vi "Tab Render.vi"(6 "Offset X (1)":i16=1, 7 "Mouse Coords":T2, 8 "error in (no error)":errorcluster, 9 "Active Idx (-1)":i32=-1, 10 "Tab Symbols":i32[](array[numeric]), 11 "Tab Names":string[](array[string])) -> (0 "error out":errorcluster, 1 "Tab X Rects":T1(array[cluster]), 2 "Tab Rects":T1(array[cluster]), 3 "Picture":picture)   [LabVIEW 2018, in "Tab.lvlib"]
uses:
  Tab.lvlib
  Theme/Theme Colors.vi
  Theme/Theme.lvlib
  <vilib>/Utility/miscctls.llb/LVPoint32TypeDef.ctl
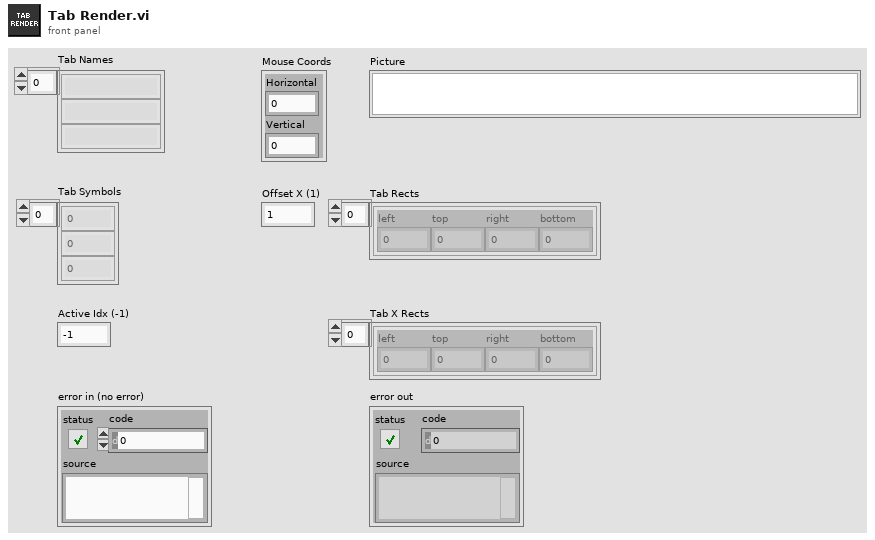
[diagram p1: front panel]
types:
  T1 = cluster{"left":i16, "top":i16, "right":i16, "bottom":i16}[]
  T2 = typedef "LVPoint32TypeDef.ctl" = cluster{"Horizontal":i32, "Vertical":i32}
  T3 = cluster{"Font Name:":string, "Size":i16, "Strikeout?":bool, "Italic?":bool, "Underline?":bool, "Outline?":bool, "Shadow?":bool, "Bold?":bool}
  T4 = enum16{"User-specified Font", "Application Font", "System Font", "Dialog Font"}
  T5 = cluster{"left":i16, "top":i16, "right":i16, "bottom":i16}
  T6 = typedef "imagedata.ctl" = cluster{"image type":i32, "image depth":i32, "image":u8[], "mask":u8[], "colors":u32[], "Rectangle":cluster{"left":i16, "top":i16, "right":i16, "bottom":i16}}
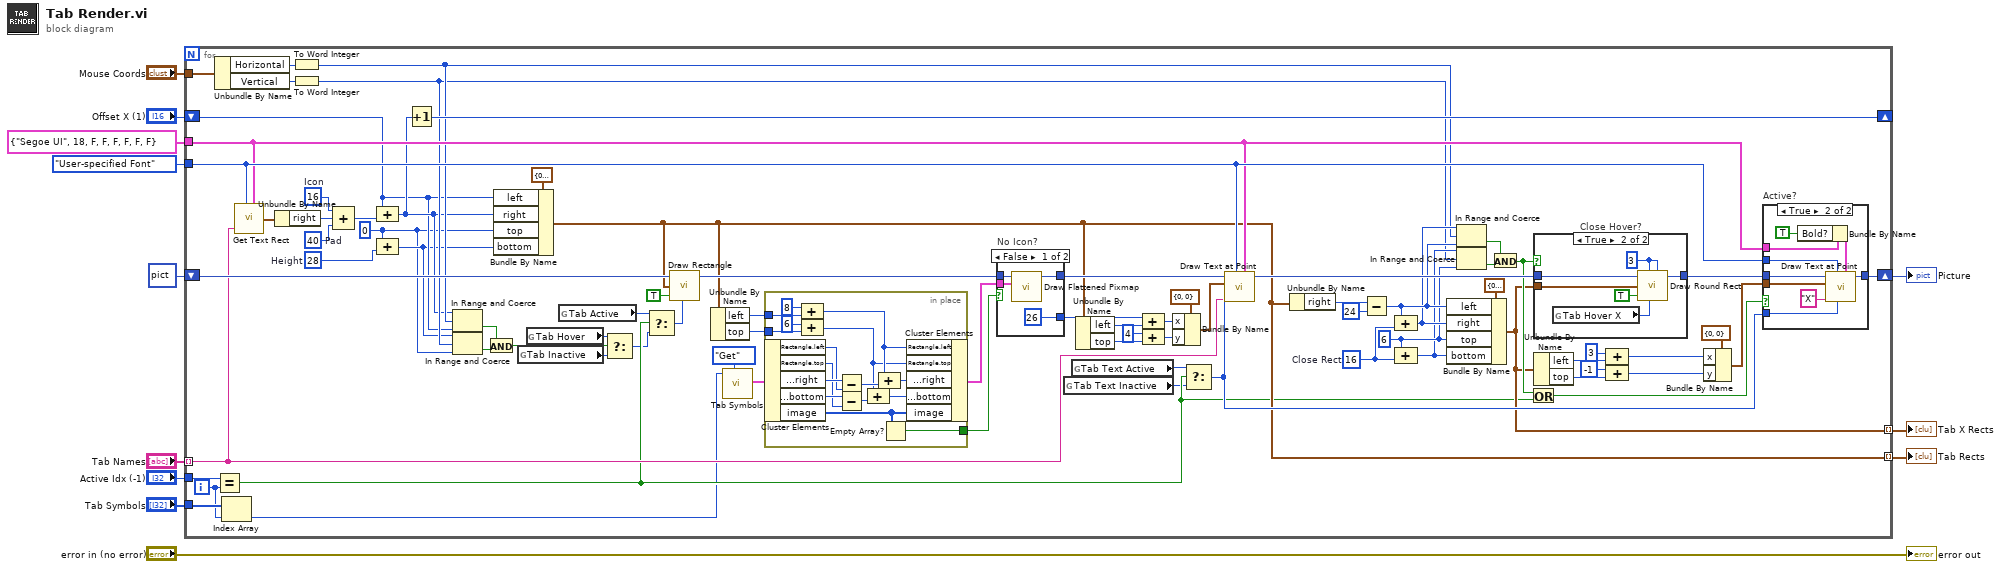
[diagram p0: block diagram]
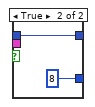
[diagram p2: hidden frame]
diagram:
  n1 = for {
    tunnel: "Tab Names" -> [w38] mode=indexing
    tunnel: T4."User-specified Font" ("desired font(Application)") -> [w50]
    tunnel: T3 {"Font Name:"="Segoe UI", "Size"=18, "Strikeout?"=FALSE, "Italic?"=FALSE, "Underline?"=FALSE, "Outline?"=FALSE, "Shadow?"=FALSE, "Bold?"=FALSE} ("[user-specified font]") -> [w49]
    shift-right: [w88] -> w2
    shift-left: picture data[5B] ("new picture") -> [w74]
    shift-right: [w82] -> _
    shift-left: "Offset X (1)" -> [w20]
    tunnel: "Mouse Coords" -> [w40]
    tunnel: [w36] -> w7 mode=indexing
    tunnel: [w35] -> w6 mode=indexing
    tunnel: "Active Idx (-1)" -> [w34]
    tunnel: "Tab Symbols" -> [w32]
    i -> [w31]
    w58 = i16 16  # Close Rect
    w42 = i16 6 ("top")
    w75 = i16 28  # Height
    w18 = i16 0 ("top")
    w78 = i16 40  # Pad
    w79 = i16 16  # Icon
    n2 = Unbundle By Name(w40) -> ("Horizontal"=w48:i32, "Vertical"=w47:i32)
    n3 = Equal?(x=w34, y=w31) -> (x = y?=w33:bool)
    n4 = Index Array(array=w32, index=w31) -> (element=w30:i32)
    n5 = call <vilib>:"Get Text Rect.vi"("desired font(Application)"=w50, "text"=w38, "[user-specified font]"=w49) -> ("rect"=w81:T5)  [unwired: 6 in]
    n6 = Unbundle By Name(w81) -> ("right"=w80:i16)
    n7 = To Word Integer(number=w48) -> (16bit integer=w23:i16)
    n8 = To Word Integer(number=w47) -> (16bit integer=w22:i16)
    n9 = Compound Arithmetic op=ADD(w79, w80, w78) -> (w76:i16)
    n10 = Compound Arithmetic op=ADD(w20, w76) -> (w21:i16)
    n11 = Compound Arithmetic op=unknown(w18, w75) -> (w19:i16)
    n12 = Increment(x=w21) -> (x+1=w82:i16)
    n13 = In Range and Coerce(upper limit=w21, x=w23, lower limit=w20) -> (In Range?=w26:bool)  [unwired: 1 out]
    n14 = In Range and Coerce(upper limit=w19, x=w22, lower limit=w18) -> (In Range?=w24:bool)  [unwired: 1 out]
    n15 = And(x=w26, y=w24) -> (x .and. y?=w25:bool)
    n16 = Bundle By Name(cluster=T5 {"left"=0, "top"=0, "right"=0, "bottom"=0} ("y"), "left"=w20, "right"=w21, "top"=w18, "bottom"=w19) -> (w36:T5)
    n17 = global read "Theme Colors.vi" "Tab Inactive"() -> (w16:u32)
    n18 = global read "Theme Colors.vi" "Tab Hover"() -> (w17:u32)
    n19 = global read "Theme Colors.vi" "Tab Active"() -> (w15:u32)
    n20 = Select(t=w17, s=w25, f=w16) -> (s? t:f=w27:u32)
    n21 = Select(t=w15, s=w33, f=w27) -> (s? t:f=w87:u32)
    n22 = call <vilib>:"Draw Rectangle.vi"("picture"=w74, "rect"=w36, "fill?(F)"=TRUE, "color(black)"=w87) -> ("new picture"=w73:picture)  [unwired: 5 in]
    n23 = Unbundle By Name(w36) -> ("left"=w70:i16, "top"=w71:i16)
    n24 = call "Tab Symbols.vi"("Action (Get)"=enum8{"Get", "Set"}."Get", "Symbol Idx"=w30) -> ("Symbol Image out"=w29:T6)  [unwired: 7 in, 2 out]
    n25 = in-place {
      in-place-border: w71 -> [w105]
      in-place-border: w70 -> [w104]
      in-place-border: [w98] -> w37
      n26 = in-place-cluster #1(w29) -> ("Rectangle.left"=w111:i16, "Rectangle.top"=w110:i16, "Rectangle.right"=w113:i16, "Rectangle.bottom"=w112:i16, "image"=w99:u8[])
      n27 = Compound Arithmetic op=ADD(i16 8 ("value"), w104) -> (w101:i16)
      n28 = Compound Arithmetic op=ADD(i16 6 ("value"), w105) -> (w100:i16)
      n29 = Subtract(x=w113, y=w111) -> (x-y=w109:i16)
      n30 = Subtract(x=w112, y=w110) -> (x-y=w106:i16)
      n31 = Compound Arithmetic op=ADD(w100, w106) -> (w107:i16)
      n32 = Compound Arithmetic op=ADD(w101, w109) -> (w108:i16)
      n33 = Empty Array?(array=w99) -> (empty?=w98:bool)
      n34 = in-place-cluster #1("Rectangle.left"=w101, "Rectangle.top"=w100, "Rectangle.right"=w108, "Rectangle.bottom"=w107, "image"=w99) -> (w72:T6)
    }
    n35 = case "No Icon?" shown="False" w37 {
      tunnel: w73 -> [w95 w97]
      tunnel: w72 -> [w94 _]
      tunnel: [i16 26 ("value") i16 8 ("value")] -> w68
      tunnel: [w92 w97] -> w62
      frame False {
        n36 = call <vilib>:"Draw Flattened Pixmap.vi"("image data"=w94, "picture"=w95) -> ("new picture"=w92:picture)  [unwired: 7 in]
      }
      frame True {
      }
    }
    n37 = global read "Theme Colors.vi" "Tab Text Inactive"() -> (w13:u32)
    n38 = global read "Theme Colors.vi" "Tab Text Active"() -> (w14:u32)
    n39 = Unbundle By Name(w36) -> ("left"=w67:i16, "top"=w66:i16)
    n40 = Compound Arithmetic op=ADD(w68, w67) -> (w65:i16)
    n41 = Compound Arithmetic op=ADD(i16 4 ("value"), w66) -> (w64:i16)
    n42 = Bundle By Name(cluster=cluster{"x":i16, "y":i16} {"x"=0, "y"=0} ("origin"), "x"=w65, "y"=w64) -> (w63:cluster{"x":i16, "y":i16})
    n43 = Select(t=w14, s=w33, f=w13) -> (s? t:f=w84:u32)
    n44 = call <vilib>:"Draw Text at Point.vi"("[user-specified font]"=w49, "text color(black)"=w84, "desired font(Application)"=w50, "text"=w38, "origin"=w63, "picture"=w62) -> ("new picture"=w89:picture)  [unwired: 4 in, 1 out]
    n45 = Unbundle By Name(w36) -> ("right"=w61:i16)
    n46 = Subtract(x=w61, y=i16 24) -> (x-y=w44:i16)
    n47 = Compound Arithmetic op=ADD(w44, w58) -> (w43:i16)
    n48 = Compound Arithmetic op=unknown(w42, w58) -> (w41:i16)
    n49 = Bundle By Name(cluster=T5 {"left"=0, "top"=0, "right"=0, "bottom"=0} ("y"), "left"=w44, "right"=w43, "top"=w42, "bottom"=w41) -> (w35:T5)
    n50 = In Range and Coerce(upper limit=w43, x=w23, lower limit=w44) -> (In Range?=w45:bool)  [unwired: 1 out]
    n51 = In Range and Coerce(upper limit=w41, x=w22, lower limit=w42) -> (In Range?=w46:bool)  [unwired: 1 out]
    n52 = And(x=w45, y=w46) -> (x .and. y?=w39:bool)
    n53 = Or(x=w39, y=w33) -> (x .or. y?=w83:bool)
    n54 = case "Close Hover?" shown="True" w39 {
      tunnel: w89 -> [w114 w120]
      tunnel: w35 -> [_ w119]
      tunnel: [w114 w118] -> w85
      frame False {
      }
      frame True {
        w116 = i16 3 ("oval width")
        n55 = global read "Theme Colors.vi" "Tab Hover X"() -> (w115:u32)
        n56 = call <vilib>:"Draw Round Rect.vi"("picture"=w120, "oval width"=w116, "rect"=w119, "fill?(F)"=TRUE, "color(black)"=w115, "oval height"=w116) -> ("new picture"=w118:picture)  [unwired: 3 in]
      }
    }
    n57 = Unbundle By Name(w35) -> ("left"=w55:i16, "top"=w54:i16)
    n58 = Compound Arithmetic op=ADD(i16 3 ("value"), w55) -> (w53:i16)
    n59 = Compound Arithmetic op=ADD(i16 -1 ("value"), w54) -> (w51:i16)
    n60 = Bundle By Name(cluster=cluster{"x":i16, "y":i16} {"x"=0, "y"=0} ("origin"), "x"=w53, "y"=w51) -> (w52:cluster{"x":i16, "y":i16})
    n61 = case "Active?" shown="True" w83 {
      tunnel: w50 -> [_ w130]
      tunnel: [w121 w129] -> w88
      tunnel: w49 -> [_ w122]
      tunnel: w52 -> [_ w127]
      tunnel: w85 -> [w121 w126]
      tunnel: w84 -> [_ w125]
      frame False {
      }
      frame True {
        n62 = Bundle By Name(cluster=w122, "Bold?"=TRUE) -> (w123:T3)
        n63 = call <vilib>:"Draw Text at Point.vi"("[user-specified font]"=w123, "text color(black)"=w125, "desired font(Application)"=w130, "text"="X", "origin"=w127, "picture"=w126) -> ("new picture"=w129:picture)  [unwired: 4 in, 1 out]
      }
    }
  }
  "Tab Rects" <- w7
  "Tab X Rects" <- w6
  "Picture" <- w2
  "error out" <- "error in (no error)"
